vi "TwosComplement (SubVI).vi"(1 "In":u16=907 format="%04x") -> (0 "Out":dbl)   [LabVIEW 2017]
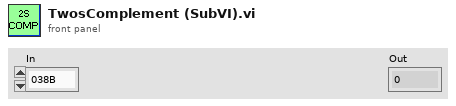
[diagram p1: front panel]
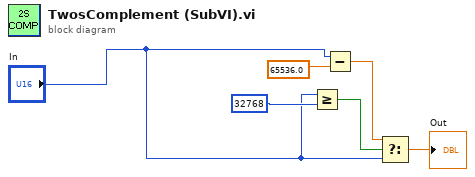
[diagram p0: block diagram]
diagram:
  n1 = Greater Or Equal?(x="In", y=u16 32768 ("Numeric")) -> (x >= y?=w6:bool)
  n2 = Subtract(x="In", y=65536.0 ("Numeric")) -> (x-y=w3:dbl)
  n3 = Select(t=w3, s=w6, f="In") -> (s? t:f=→"Out":dbl)
